vi "obj_DataLog Expression Update Timing.vi"(0 "method":T1, 9 "tag index":i32, 11 "period (ms)":u16) -> (4 "available? {next due}":bool, 10 "tag index out":i32)   [LabVIEW 2012]
doc: "This object serves to time the periodic update of expressions with little overhead."
uses:
  typedefs/t_DataLog Expression Update Timing Methods.ctl
  subvis/private/glb_DataLog Runtime Parameterisation.vi
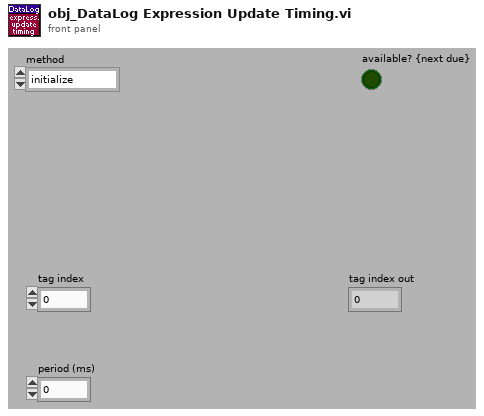
[diagram p1: front panel]
types:
  T1 = typedef "t_DataLog Expression Update Timing Methods.ctl" = enum16{"initialize", "schedule", "make due", "next due", "cleanup"}
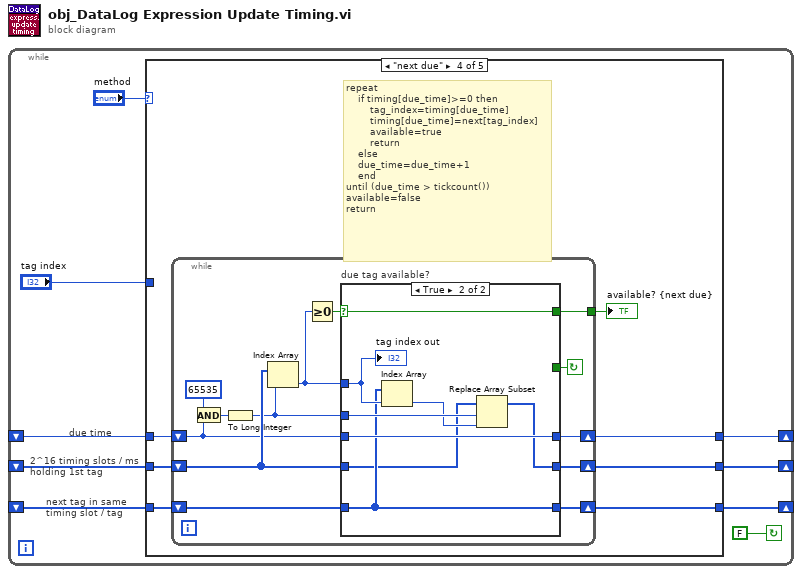
[diagram p0: block diagram]
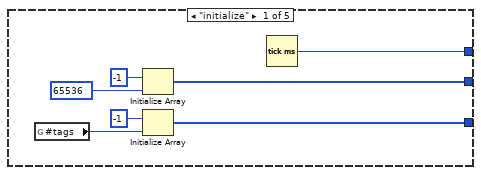
[diagram p2: hidden frame]
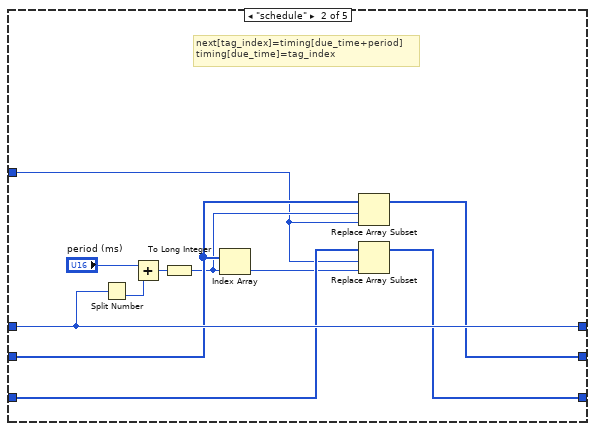
[diagram p3: hidden frame]
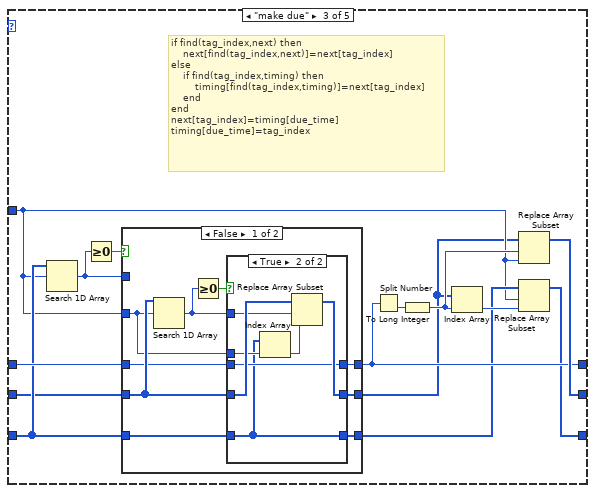
[diagram p4: hidden frame]
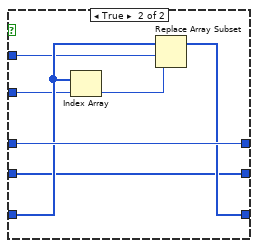
[diagram p6: hidden frame]
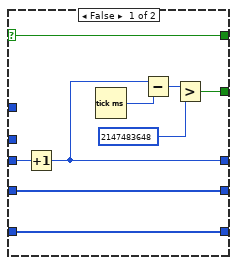
[diagram p7: hidden frame]
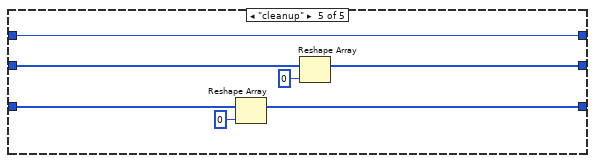
[diagram p8: hidden frame]
diagram:
  n1 = while {
    shift-right: [w7] -> _
    shift-left: _ -> [w6]
    shift-right: [w4] -> _
    shift-left: _ -> [w5]
    shift-right: [w2] -> _
    shift-left: _ -> [w3]
    stop <- FALSE continue-if-true
    # "next tag in same\ntiming slot / tag"
    # "2^16 timing slots / ms\nholding 1st tag"
    # "due time"
    n2 = case shown="\"next due\"" "method" {
      tunnel: w6 -> [_ w27 w35 w70 w105]
      tunnel: [w14 w27 w34 w69 w105] -> w7
      tunnel: w5 -> [_ w20 w29 w72 w109]
      tunnel: [w12 w19 w40 w71 w106] -> w4
      tunnel: w3 -> [_ w23 w33 w74 w108]
      tunnel: [w15 w22 w32 w73 w107] -> w2
      tunnel: "tag index" -> [_ w17 w30 _ _]
      frame "initialize" {
        n3 = global read "glb_DataLog Runtime Parameterisation.vi" "#tags"() -> (w10:i32)
        n4 = Initialize Array(-1, 65536 ("dimension size")) -> (w12:i32[])
        n5 = Initialize Array(-1, w10) -> (w15:i32[])
        n6 = Tick Count (ms)() -> (millisecond timer value=w14:u32)
      }
      frame "schedule" {
        # "next[tag_index]=timing[due_time+period]\ntiming[due_time]=tag_index"
        n7 = Split Number(x=w27) -> (lo(x)=w26:u16)  [unwired: 1 out]
        n8 = Add(x="period (ms)", y=w26) -> (x+y=w24:u16)
        n9 = To Long Integer(number=w24) -> (32bit integer=w18:i32)
        n10 = Index Array(array=w20, index=w18) -> (element=w21:i32)
        n11 = Replace Array Subset(array=w20, new element=w17, index=w18) -> (w19:i32[])
        n12 = Replace Array Subset(array=w23, new element=w21, index=w17) -> (w22:i32[])
      }
      frame "make due" {
        # "if find(tag_index,next) then\n    next[find(tag_index,next)]=next[tag_index]\nelse\n    if find(tag_index,timing) then\n        timing[find(tag_index,timing)]=next[tag_index]\n    end\nend\nnext[tag_index]=timing[due_time]\ntiming[due_time]=tag_index"
        n13 = Search 1D Array(1D array=w33, element=w30) -> (index of element=w36:i32)  [unwired: 1 in]
        n14 = Greater Or Equal To 0?(x=w36) -> (x >= 0?=w37:bool)
        n15 = case shown="False" w37 {
          tunnel: w36 -> [_ w65]
          tunnel: w35 -> [w42 w67]
          tunnel: [w43 w67] -> w34
          tunnel: w33 -> [w49 w66]
          tunnel: [w48 w64] -> w31
          tunnel: w30 -> [w45 w62]
          tunnel: [w44 w61] -> w28
          tunnel: w29 -> [w46 w61]
          frame False {
            n16 = Search 1D Array(1D array=w46, element=w45) -> (index of element=w47:i32)  [unwired: 1 in]
            n17 = Greater Or Equal To 0?(x=w47) -> (x >= 0?=w50:bool)
            n18 = case shown="True" w50 {
              tunnel: w49 -> [w51 w54]
              tunnel: [w51 w54] -> w48
              tunnel: w46 -> [w52 w59]
              tunnel: w47 -> [_ w58]
              tunnel: w45 -> [_ w57]
              tunnel: [w52 w56] -> w44
              tunnel: w42 -> [w53 w55]
              tunnel: [w53 w55] -> w43
              frame False {
              }
              frame True {
                n19 = Index Array(array=w54, index=w57) -> (element=w60:i32)
                n20 = Replace Array Subset(array=w59, new element=w60, index=w58) -> (w56:i32[])
              }
            }
          }
          frame True {
            n21 = Index Array(array=w66, index=w62) -> (element=w63:i32)
            n22 = Replace Array Subset(array=w66, new element=w63, index=w65) -> (w64:i32[])
          }
        }
        n23 = Split Number(x=w34) -> (lo(x)=w39:u16)  [unwired: 1 out]
        n24 = To Long Integer(number=w39) -> (32bit integer=w38:i32)
        n25 = Index Array(array=w28, index=w38) -> (element=w41:i32)
        n26 = Replace Array Subset(array=w28, new element=w30, index=w38) -> (w40:i32[])
        n27 = Replace Array Subset(array=w31, new element=w41, index=w30) -> (w32:i32[])
      }
      frame "next due" {
        # "repeat\n    if timing[due_time]>=0 then\n        tag_index=timing[due_time]\n        timing[due_time]=next[tag_index]\n        available=true\n        return\n    else\n    due_time=due_time+1\n    end\nuntil (due_time > tickcount())\navailable=false\nreturn"
        n28 = while {
          shift-right: [w81] -> w73
          shift-left: w74 -> [w83]
          shift-right: [w82] -> w71
          shift-left: w72 -> [w79]
          shift-right: [w84] -> w69
          shift-left: w70 -> [w78]
          tunnel: [w75] -> w68
          stop <- w85 continue-if-true
          n29 = And(x=u32 65535 ("dimension size"), y=w78) -> (x .and. y?=w77:u32)
          n30 = To Long Integer(number=w77) -> (32bit integer=w76:i32)
          n31 = Index Array(array=w79, index=w76) -> (element=w80:i32)
          n32 = Greater Or Equal To 0?(x=w80) -> (x >= 0?=w86:bool)
          n33 = case "due tag available?" shown="True" w86 {
            selector: w86 -> [w88 w100]
            tunnel: w78 -> [w96 w102]
            tunnel: [w93 _] -> w85
            tunnel: [w90 w102] -> w84
            tunnel: w83 -> [w91 w99]
            tunnel: w79 -> [w92 w98]
            tunnel: [w92 w97] -> w82
            tunnel: [w91 w99] -> w81
            tunnel: w80 -> [_ w101]
            tunnel: w76 -> [_ w104]
            tunnel: [w88 w100] -> w75
            frame False {
              n34 = Increment(x=w96) -> (x+1=w90:u32)
              n35 = Tick Count (ms)() -> (millisecond timer value=w89:u32)
              n36 = Subtract(x=w90, y=w89) -> (x-y=w95:u32)
              n37 = Greater?(x=w95, y=u32 2147483648 ("dimension size")) -> (0:w93:bool)
            }
            frame True {
              n38 = Index Array(array=w99, index=w101) -> (element=w103:i32)
              n39 = Replace Array Subset(array=w98, new element=w103, index=w104) -> (w97:i32[])
              "tag index out" <- w101
            }
          }
        }
        "available? {next due}" <- w68
      }
      frame "cleanup" {
        n40 = Reshape Array(w108, 0 ("dimension size")) -> (w107:i32[])
        n41 = Reshape Array(w109, 0 ("dimension size")) -> (w106:i32[])
      }
    }
  }
